vi "read2002.vi"(8 "error in (no error)":errorcluster, 9 "function (Vdc:1)":u16(ring)=1 items=["ac voltage", "dc voltage", "2-wire resistance", "4-wire resistance", "ac current", "dc current", "frequency", "temperature"]) -> (0 "error out":errorcluster, 1 "medicion":dbl, 2 "Reading Result":string)   [LabVIEW 2019, in "K2002_GPIB.lvlib"]
uses:
  K2002_GPIB.lvlib
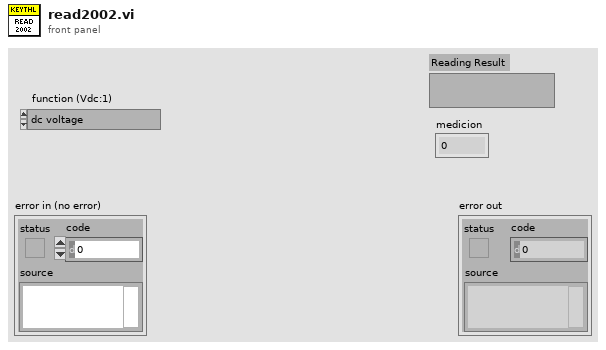
[diagram p1: front panel]
types:
  T1 = cluster{"error":bool, "code":i32, "source":string}
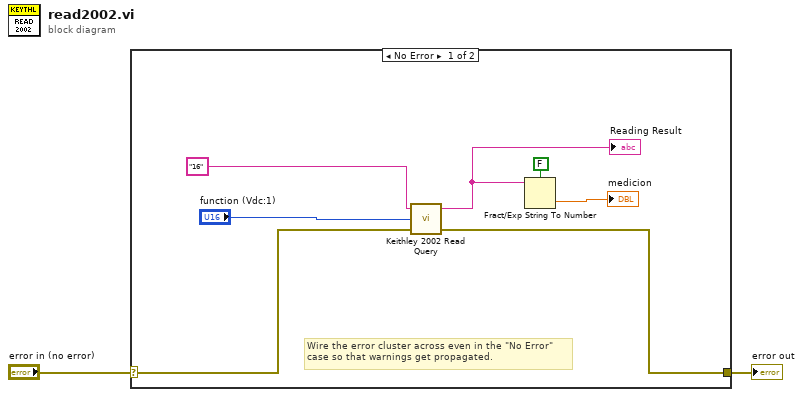
[diagram p0: block diagram]
diagram:
  n1 = case shown="No Error" "error in (no error)" {
    selector: "error in (no error)" -> [w7 w10]
    tunnel: [w6 w10] -> w1
    frame No Error {
      # "Wire the error cluster across even in the \"No Error\"\ncase so that warnings get propagated."
      n2 = call <instrlib>:"Keithley 2002 Read Query.vi"("error in"=w7, "function (Vdc:1)"="function (Vdc:1)", "GPIB Address"="16") -> ("error out"=w6:T1, "Reading Result"=w5:string)  [unwired: 1 in]
      "Reading Result" <- w5
      n3 = Fract/Exp String To Number(use system decimal point (T)=FALSE, string=w5) -> (number=→"medicion":dbl)  [unwired: 2 in, 1 out]
    }
    frame Error {
    }
  }
  "error out" <- w1
